vi "TC110_NoFGV.vi"(7 "Function":T3=enum."Read command", 8 "Error in":errorcluster, 10 "Settings in":T2) -> (0 "Error out":errorcluster, 1 "Status_string":string, 2 "Settings out":T2, 3 "output cluster":T1)   [LabVIEW 2018]
uses:
  Ctl/Function_of_TC110.ctl
  PublicSubVI/Ctl/_ctl_RT_TurboSettings.ctl
  Example/RS485_TurboPump/Public/Turbopumps/PV Operating adjustment - Cluster.ctl
  Example/RS485_TurboPump/Pfeiffer Vacuum.lvlib
panel:
  in  "VISA session":refnum<visa-resource-name>
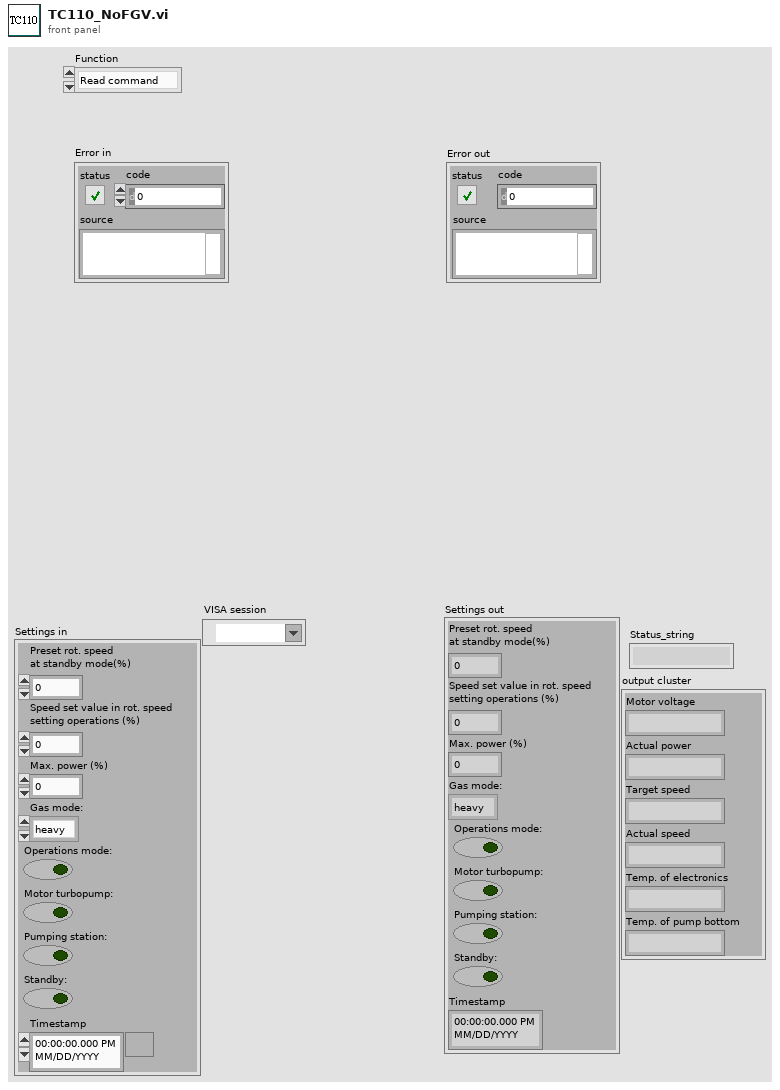
[diagram p1: front panel]
types:
  T1 = cluster{"Motor voltage":string, "Actual power":string, "Target speed":string, "Actual speed":string, "Temp. of electronics":string, "Temp. of pump bottom":string}
  T2 = typedef "_ctl_RT_TurboSettings.ctl" = cluster{"Preset rot. speed \nat standby mode(%)":dbl, "Speed set value in rot. speed \nsetting operations (%)":dbl, "Max. power (%)":dbl, "Gas mode: ":enum16{"heavy", "light", "helium"}, "Operations mode: ":bool, "Motor turbopump: ":bool, "Pumping station: ":bool, "Standby: ":bool, "Timestamp":timestamp}
  T3 = typedef "Function_of_TC110.ctl" = enum16{"Initialisation", "Read status", "Write command", "Read command"}
  T4 = typedef "Pfeiffer Vacuum.lvlib/PV Operating adjustment - Cluster.ctl" = cluster{"Parameter":u16, "Parameter\nread only<->describe":bool, "off<->on":bool, "Rotation speed set value\nin rot. speed setting\noperations [%]":dbl, "Preset rotation Speed\nat Standby mode (%)":dbl, "maximum power\nsetpoint [%]":i32, "Gas mode":u16}
  T5 = enum16{"temperature inverter [°C] (324)", "temperature electronic [°C] (326)", "temperature pump bottom [°C] (330)", "temperature bearing [°C] (342)", "temperature motor [°C] (346)", "temperature rotor [°C] (384)"}
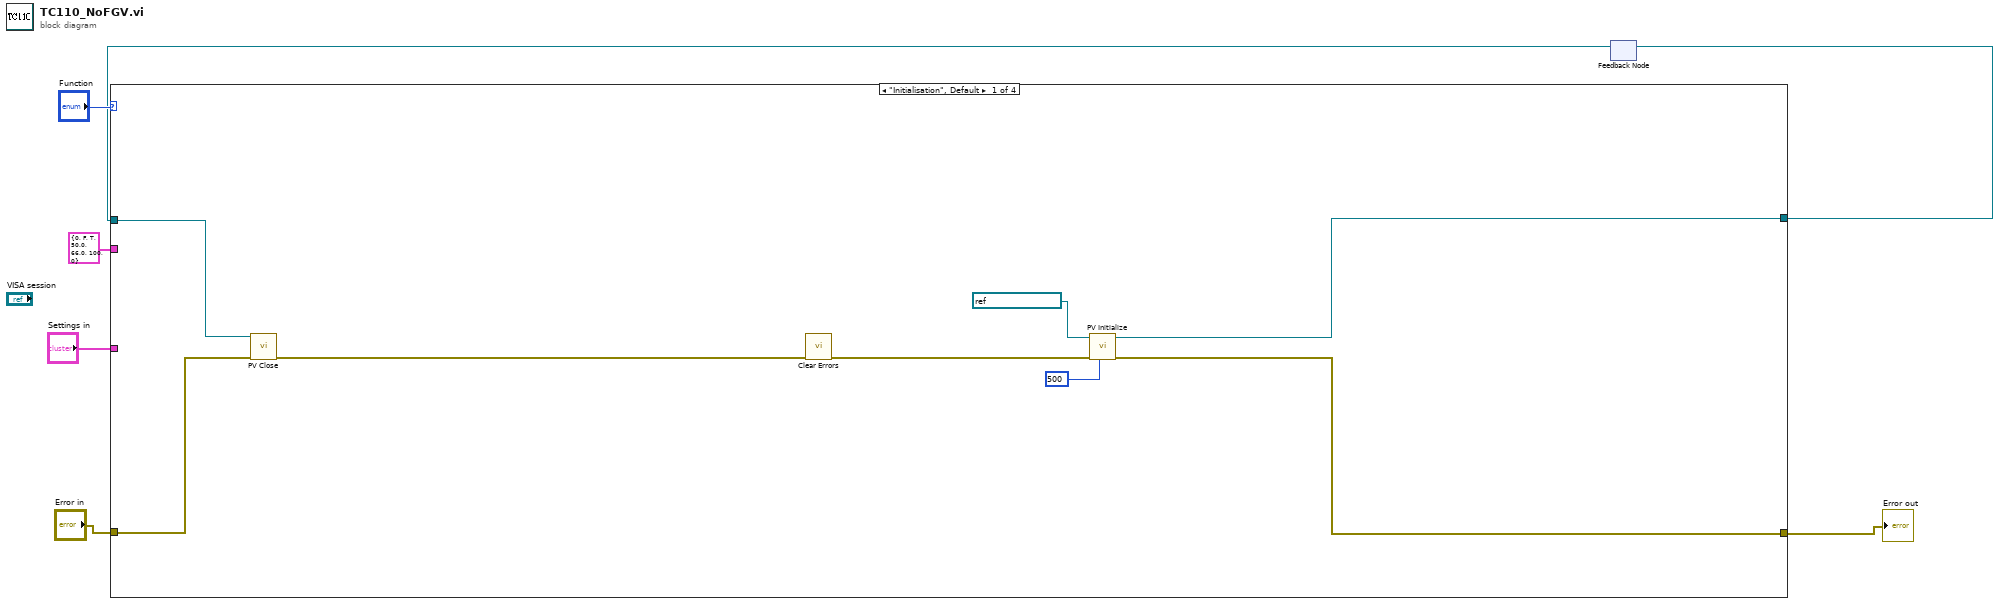
[diagram p0: block diagram]
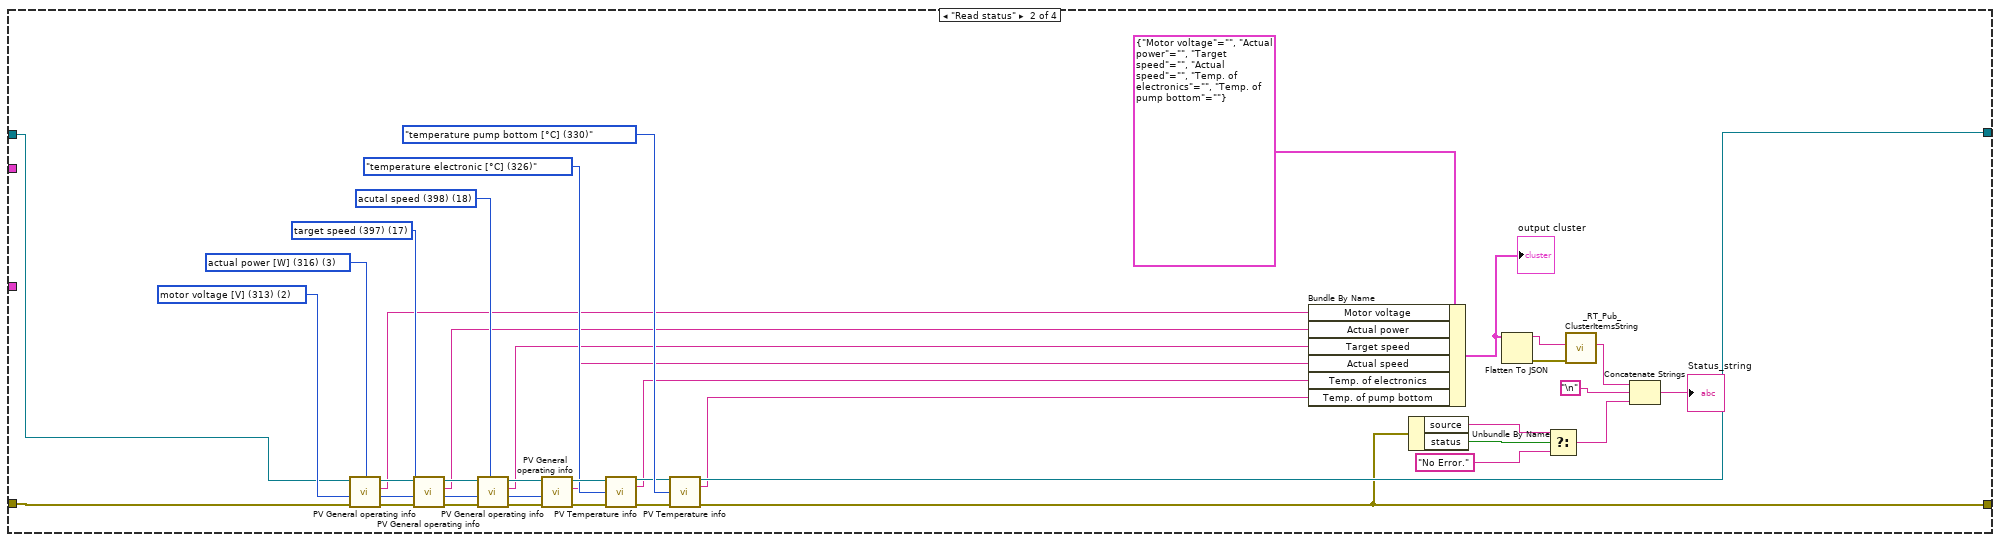
[diagram p2: hidden frame]
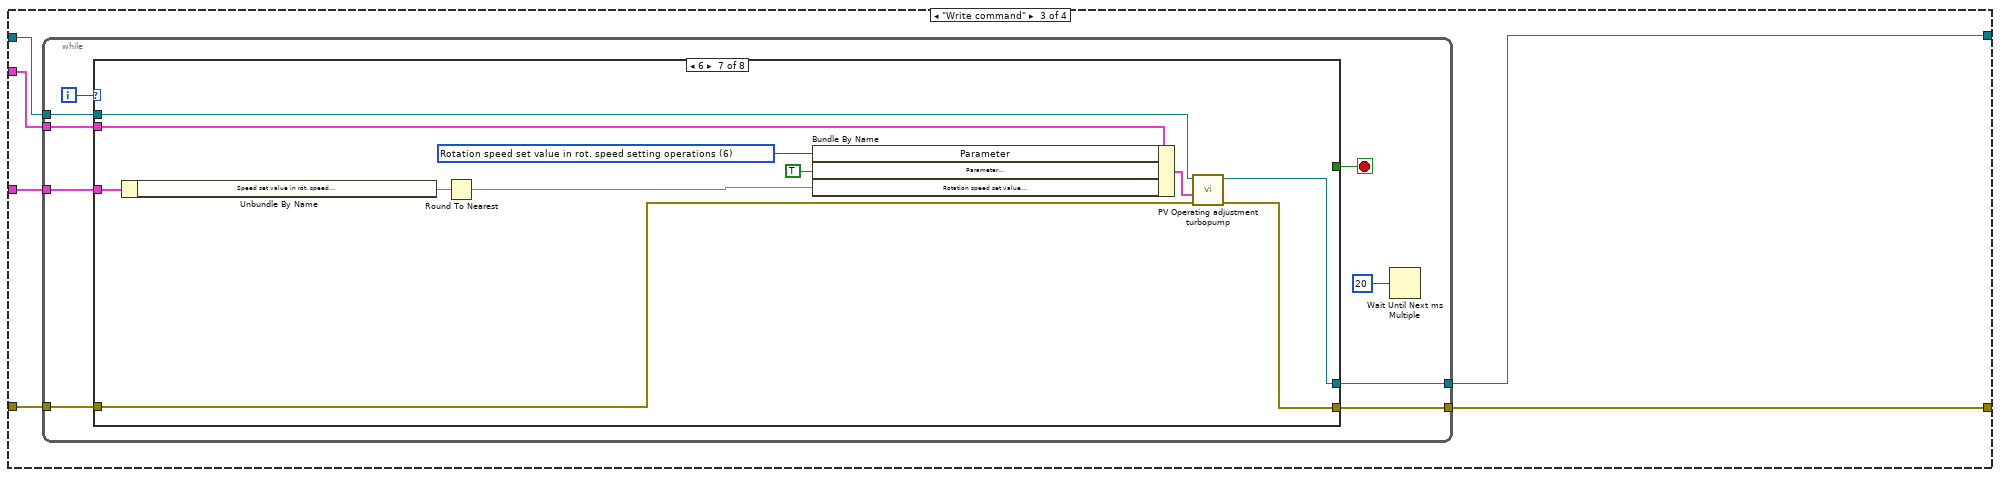
[diagram p3: hidden frame]
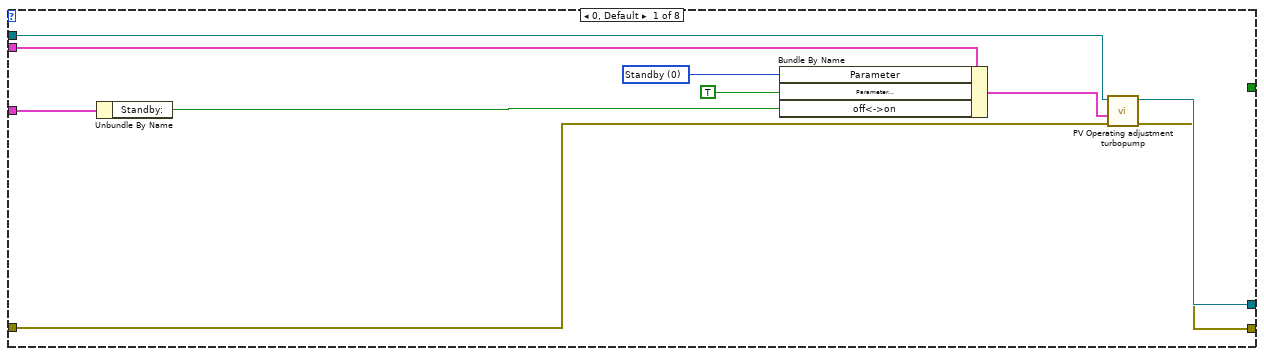
[diagram p4: hidden frame]
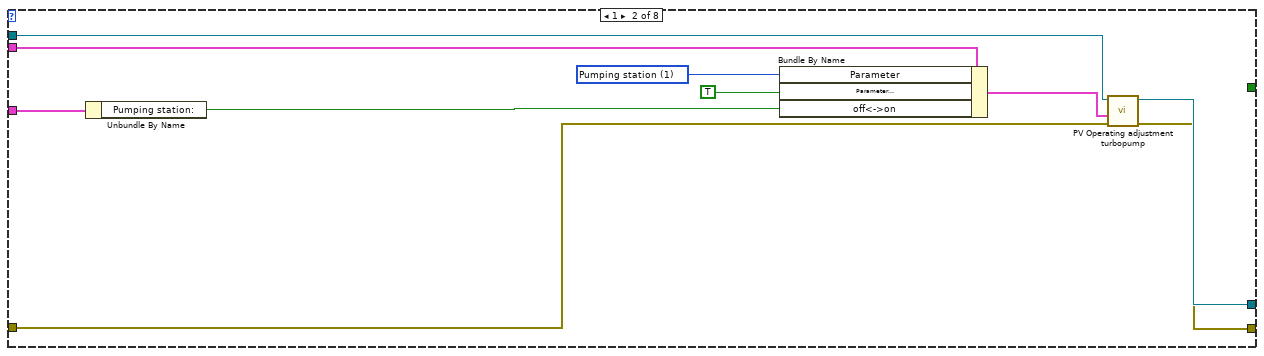
[diagram p5: hidden frame]
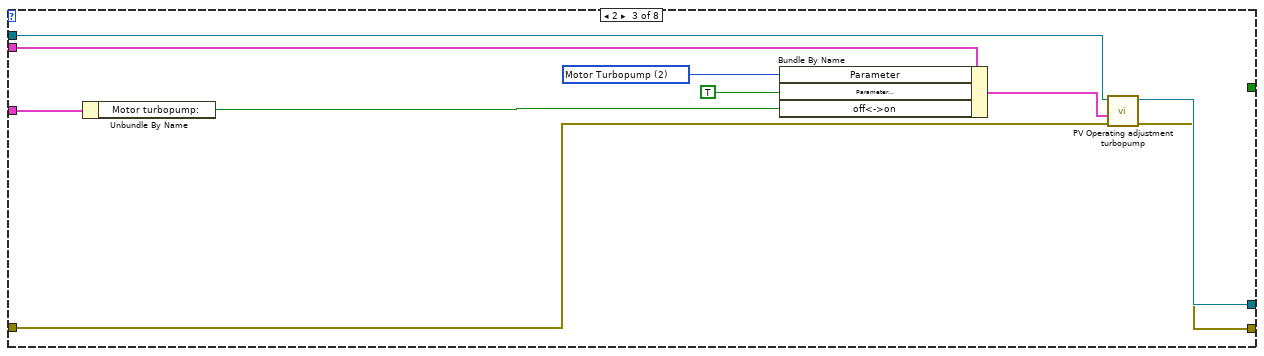
[diagram p6: hidden frame]
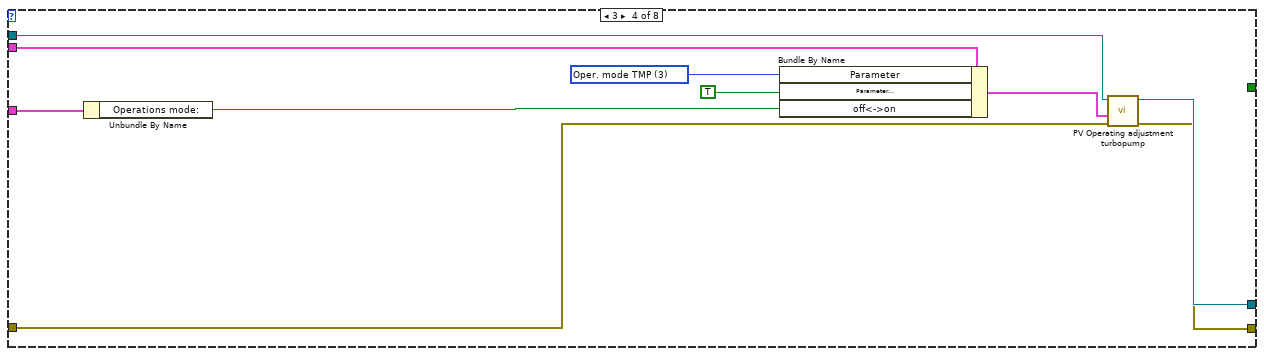
[diagram p7: hidden frame]
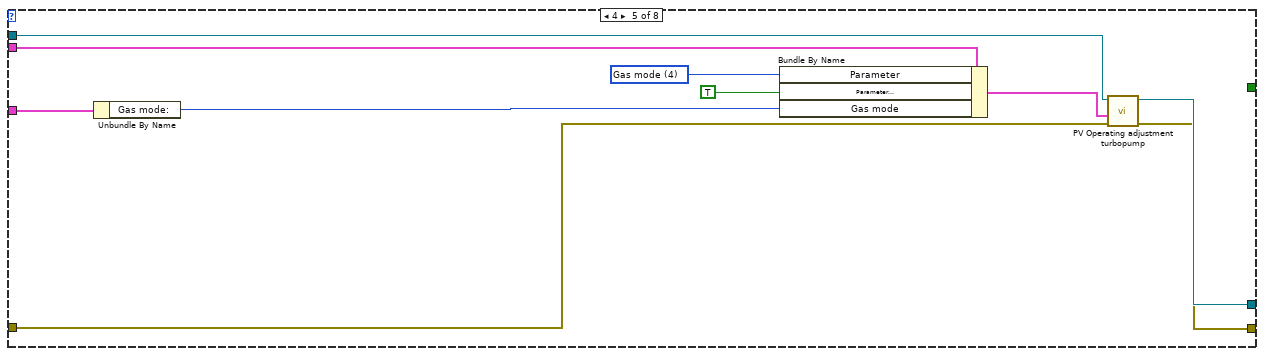
[diagram p8: hidden frame]
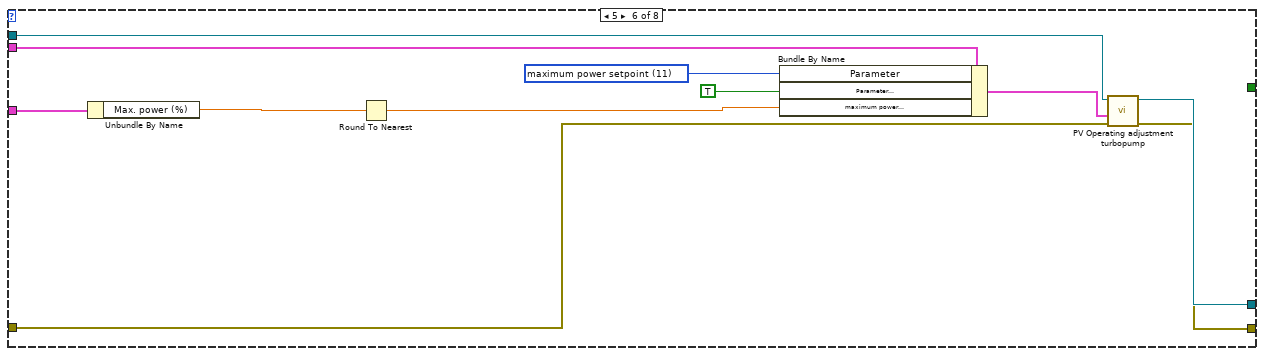
[diagram p9: hidden frame]
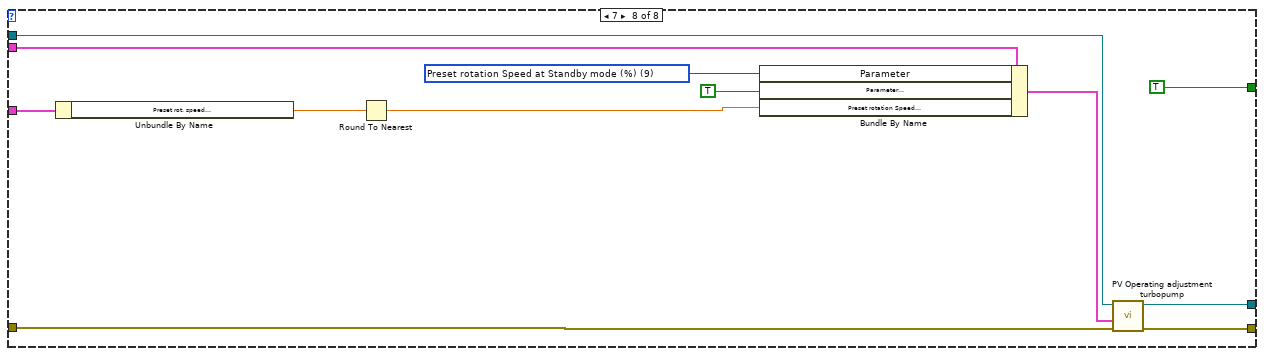
[diagram p10: hidden frame]
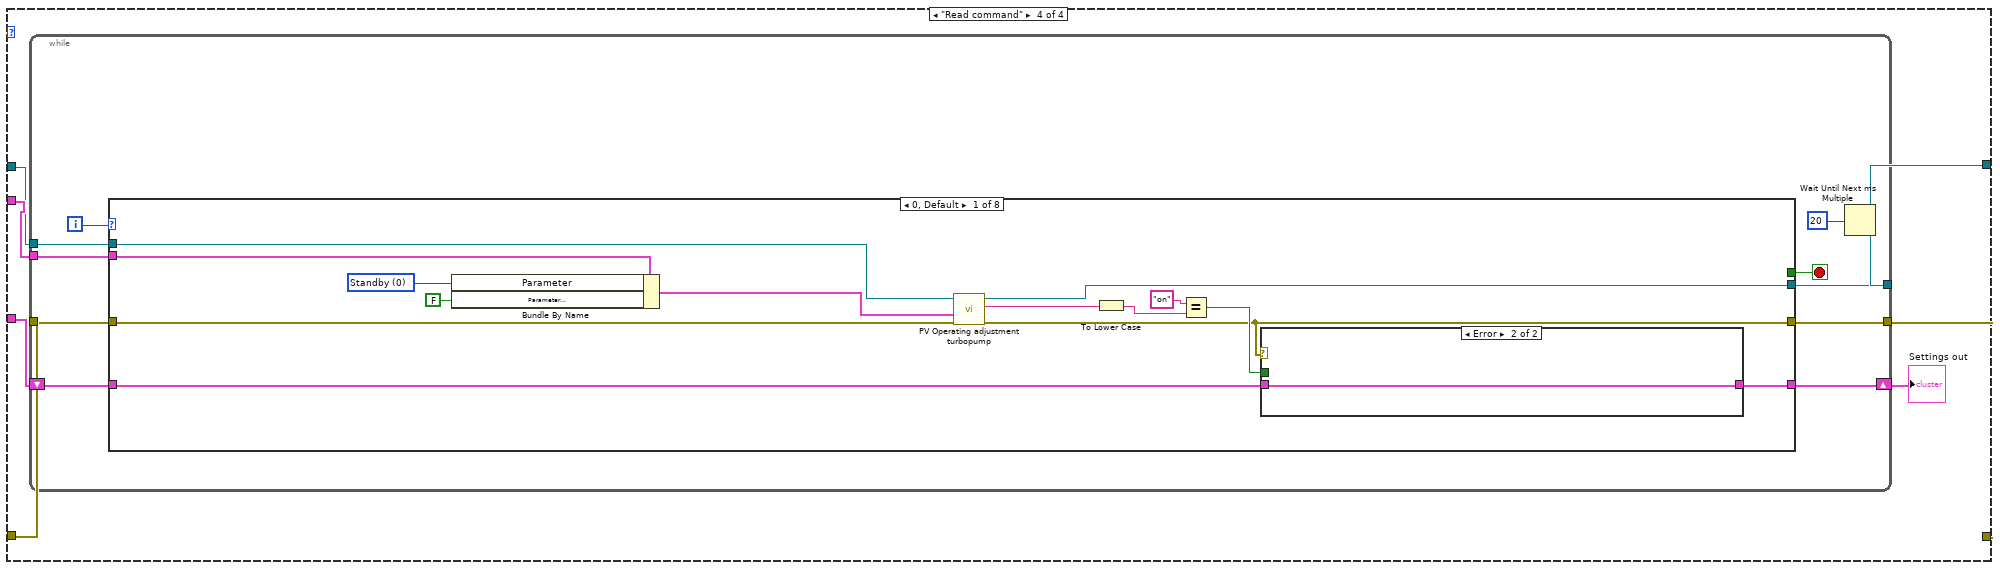
[diagram p11: hidden frame]
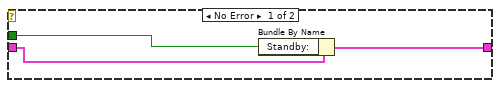
[diagram p12: hidden frame]
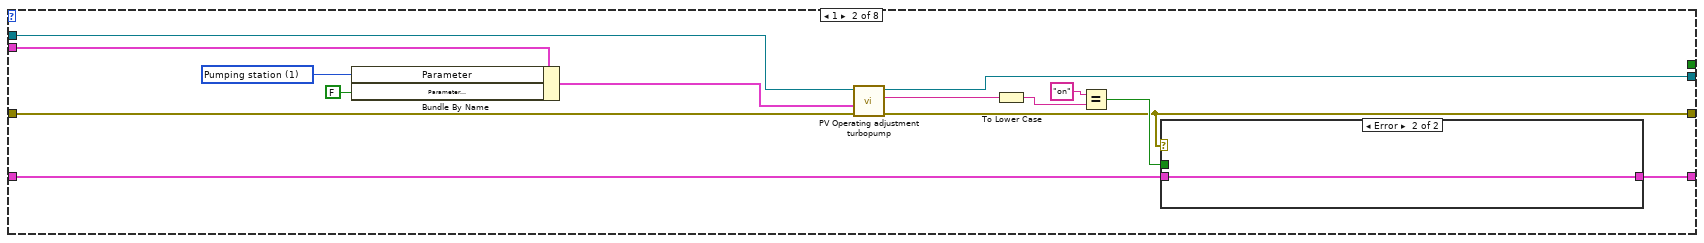
[diagram p13: hidden frame]
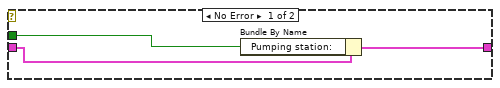
[diagram p14: hidden frame]
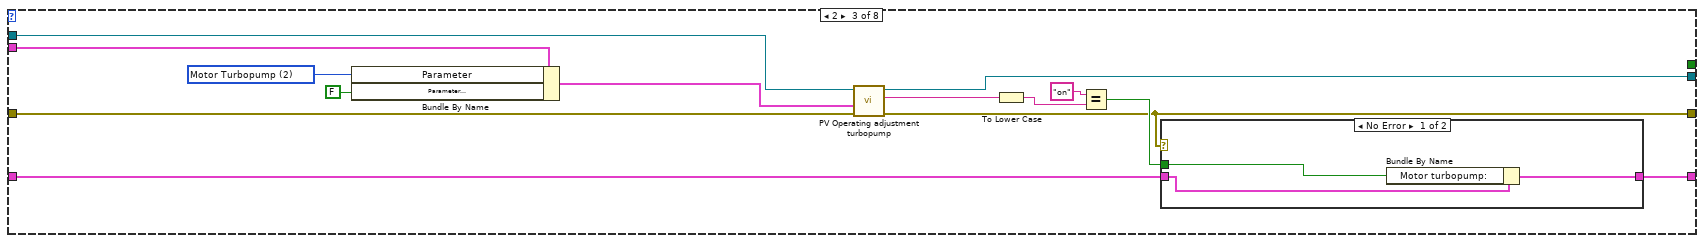
[diagram p15: hidden frame]
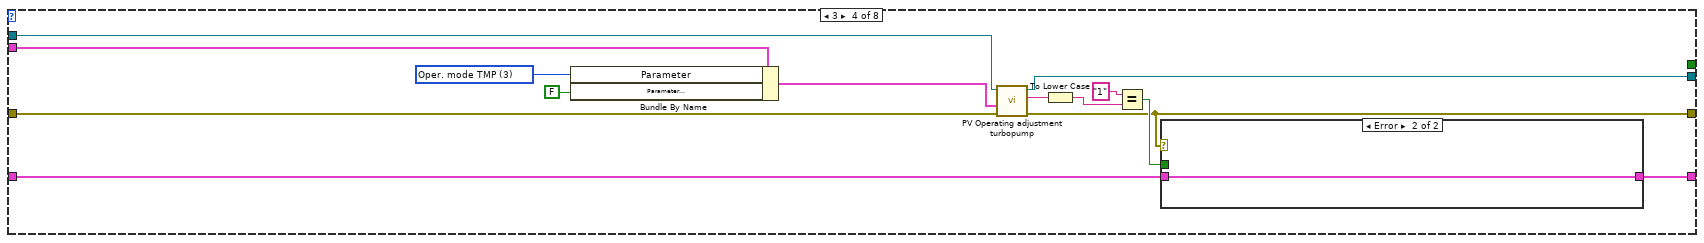
[diagram p17: hidden frame]
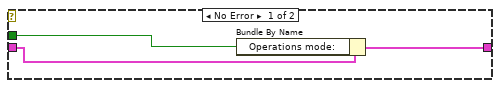
[diagram p18: hidden frame]
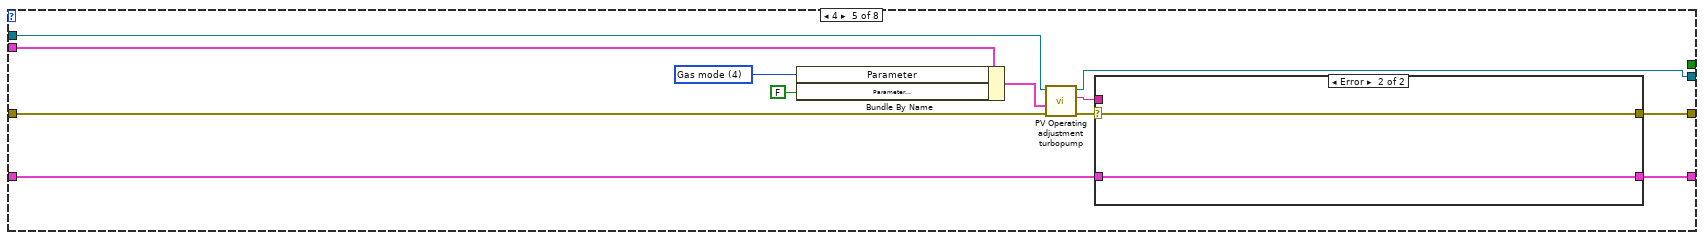
[diagram p19: hidden frame]
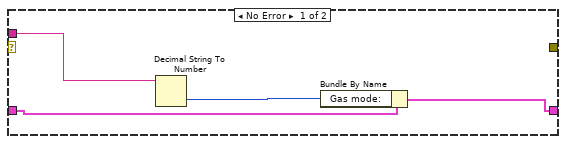
[diagram p20: hidden frame]
diagram:
  n1 = feedback #1() -> (w4:refnum<visa-resource-name>)  [unwired: 1 in]
  n2 = case shown="\"Initialisation\", Default" "Function" {
    tunnel: "Error in" -> [w11 w16 w55 w154]
    tunnel: [w14 w32 w54 w158] -> w5
    tunnel: w4 -> [w12 w17 w56 w155]
    tunnel: [w13 w25 w53 w157] -> w3
    tunnel: "Settings in" -> [_ _ w58 w153]
    tunnel: T4 {"Parameter"=0, "Parameter\nread only<->describe"=FALSE, "off<->on"=TRUE, "Rotation speed set value\nin rot. speed setting\noperations [%]"=50.0, "Preset rotation Speed\nat Standby mode (%)"=66.0, "maximum power\nsetpoint [%]"=100, "Gas mode"=0} ("Operating adjustment - Cluster") -> [_ _ w57 w156]
    frame "Initialisation", Default {
      n3 = call "PV Close.vi"("VISA session"=w12, "error in (no error)"=w11) -> ("error out"=w10:errorcluster)  [unwired: 13 in]
      n4 = call <vilib>:"Clear Errors.vi"("error in (no error)"=w10) -> ("error out"=w9:errorcluster)  [unwired: 5 in, 1 out]
      n5 = call "PV Initialize.vi"("Timeout Value"=u32 500, "error in (no error)"=w9, "VISA session in"=refnum<visa-resource-name> "ASRL3::INSTR") -> ("error out"=w13:errorcluster, "VISA session out"=w14:refnum<visa-resource-name>)  [unwired: 7 in]
    }
    frame "Read status" {
      w48 = u16 18 items=["nominal speed [Hz] (default) (315)", "intermediate circut current [A] (310)", "motor voltage [V] (313)", "actual power [W] (316)", "operating hours pump [h] (311)", "operating hours drive [h] (314)", "pump cycles (read only) (319)", "status oil sensor (read only) (301)", "speed switchpoint attained (read only) (302)", "overtemperature drive (read only) (304)", "overtemperature pump (read only) (305)", "target speed attained (read only) (306)", "pump accelerates (read only) (307) ", "controlled by remote (300)", "motor phase current [A] (317)", "acceleration / deceleration [rm/s] (336)", "hardware version controller (354)", "target speed (397)", "acutal speed (398)", "nominal speed (399)", "software version control unit (read only) (352)"] ("Parameter")
      w49 = u16 17 items=["nominal speed [Hz] (default) (315)", "intermediate circut current [A] (310)", "motor voltage [V] (313)", "actual power [W] (316)", "operating hours pump [h] (311)", "operating hours drive [h] (314)", "pump cycles (read only) (319)", "status oil sensor (read only) (301)", "speed switchpoint attained (read only) (302)", "overtemperature drive (read only) (304)", "overtemperature pump (read only) (305)", "target speed attained (read only) (306)", "pump accelerates (read only) (307) ", "controlled by remote (300)", "motor phase current [A] (317)", "acceleration / deceleration [rm/s] (336)", "hardware version controller (354)", "target speed (397)", "acutal speed (398)", "nominal speed (399)", "software version control unit (read only) (352)"] ("Parameter")
      w50 = u16 3 items=["nominal speed [Hz] (default) (315)", "intermediate circut current [A] (310)", "motor voltage [V] (313)", "actual power [W] (316)", "operating hours pump [h] (311)", "operating hours drive [h] (314)", "pump cycles (read only) (319)", "status oil sensor (read only) (301)", "speed switchpoint attained (read only) (302)", "overtemperature drive (read only) (304)", "overtemperature pump (read only) (305)", "target speed attained (read only) (306)", "pump accelerates (read only) (307) ", "controlled by remote (300)", "motor phase current [A] (317)", "acceleration / deceleration [rm/s] (336)", "hardware version controller (354)", "target speed (397)", "acutal speed (398)", "nominal speed (399)", "software version control unit (read only) (352)"] ("Parameter")
      w52 = u16 2 items=["nominal speed [Hz] (default) (315)", "intermediate circut current [A] (310)", "motor voltage [V] (313)", "actual power [W] (316)", "operating hours pump [h] (311)", "operating hours drive [h] (314)", "pump cycles (read only) (319)", "status oil sensor (read only) (301)", "speed switchpoint attained (read only) (302)", "overtemperature drive (read only) (304)", "overtemperature pump (read only) (305)", "target speed attained (read only) (306)", "pump accelerates (read only) (307) ", "controlled by remote (300)", "motor phase current [A] (317)", "acceleration / deceleration [rm/s] (336)", "hardware version controller (354)", "target speed (397)", "acutal speed (398)", "nominal speed (399)", "software version control unit (read only) (352)"] ("Parameter")
      n6 = call "PV General operating info.vi"("error in (no error)"=w16, "Parameter"=w52, "VISA session"=w17) -> ("error out"=w45:errorcluster, "response (data)"=w35:string, "dup VISA session"=w51:refnum<visa-resource-name>)  [unwired: 6 in]
      n7 = call "PV General operating info.vi"("error in (no error)"=w45, "Parameter"=w50, "VISA session"=w51) -> ("error out"=w44:errorcluster, "response (data)"=w29:string, "dup VISA session"=w47:refnum<visa-resource-name>)  [unwired: 6 in]
      n8 = call "PV General operating info.vi"("error in (no error)"=w44, "Parameter"=w49, "VISA session"=w47) -> ("error out"=w43:errorcluster, "response (data)"=w30:string, "dup VISA session"=w46:refnum<visa-resource-name>)  [unwired: 6 in]
      n9 = call "PV General operating info.vi"("error in (no error)"=w43, "Parameter"=w48, "VISA session"=w46) -> ("error out"=w39:errorcluster, "response (data)"=w34:string, "dup VISA session"=w42:refnum<visa-resource-name>)  [unwired: 6 in]
      n10 = call "PV Temperature info.vi"("VISA session"=w42, "Parameter"=T5."temperature electronic [°C] (326)", "error in (no error)"=w39) -> ("dup VISA session"=w38:refnum<visa-resource-name>, "response (data)"=w33:string, "error out"=w37:errorcluster)  [unwired: 10 in]
      n11 = call "PV Temperature info.vi"("VISA session"=w38, "Parameter"=T5."temperature pump bottom [°C] (330)", "error in (no error)"=w37) -> ("dup VISA session"=w32:refnum<visa-resource-name>, "response (data)"=w31:string, "error out"=w25:errorcluster)  [unwired: 10 in]
      n12 = Bundle By Name(cluster=T1 {"Motor voltage"="", "Actual power"="", "Target speed"="", "Actual speed"="", "Temp. of electronics"="", "Temp. of pump bottom"=""}, "Motor voltage"=w35, "Actual power"=w29, "Target speed"=w30, "Actual speed"=w34, "Temp. of electronics"=w33, "Temp. of pump bottom"=w31) -> (w28:T1)
      "output cluster" <- w28
      n13 = Unbundle By Name(w25) -> ("source"=w23:string, "status"=w24:bool)
      n14 = Flatten To JSON(anything=w28) -> (JSON string=w27:string, 11:w26:errorcluster)  [unwired: 2 in]
      n15 = Select(t=w23, s=w24, f="No Error.") -> (s? t:f=w19:string)
      n16 = call "_RT_Pub_ClusterItemsString.vi"("error in (no error)"=w26, "JSON string"=w27) -> ("result string"=w21:string)  [unwired: 8 in, 1 out]
      n17 = Concatenate Strings(w21, "\n" ("string"), w19) -> (→"Status_string":string)
    }
    frame "Write command" {
      n18 = while {
        tunnel: w58 -> [w67]
        tunnel: w56 -> [w63]
        tunnel: w55 -> [w61]
        tunnel: [w64] -> w54
        tunnel: [w62] -> w53
        tunnel: w57 -> [w66]
        i -> [w65]
        stop <- w60 stop-if-true
        n19 = case shown="6" w65 {
          tunnel: w67 -> [w75 w85 w95 w105 w115 w126 w137 w149]
          tunnel: w66 -> [w77 w87 w97 w107 w117 w128 w139 w151]
          tunnel: [w73 w83 w93 w103 w113 w124 w135 w147] -> w64
          tunnel: w63 -> [w72 w82 w92 w102 w112 w123 w134 w146]
          tunnel: [w70 w80 w90 w100 w110 w121 w132 w145] -> w62
          tunnel: w61 -> [w69 w79 w89 w99 w109 w120 w131 w144]
          tunnel: [_ _ _ _ _ _ _ TRUE] -> w60
          frame 0, Default {
            w68 = u16 0 items=[" Standby", " Pumping station", " Motor Turbopump", " Oper. mode TMP", " Gas mode", " Operating mode drive unit", " Rotation speed set value in rot. speed setting operations", " Set rotation speed TMP [Hz] (read only)", " Actual rotation speed TMP [Hz] (read only)", " Preset rotation Speed at Standby mode (%)", " Max. rotations speed ", " maximum power setpoint"] ("Parameter")
            n20 = Unbundle By Name(w75) -> ("Standby:"=w74:bool)
            n21 = Bundle By Name(cluster=w77, "Parameter"=w68, "Parameter\nread only<->describe"=TRUE ("Parameter\nread only<->describe"), "off<->on"=w74) -> (w71:T4)
            n22 = call "PV Operating adjustment turbopump.vi"("error in (no error)"=w69, "Operating adjustment - Cluster"=w71, "VISA session"=w72) -> ("error out"=w70:errorcluster, "dup VISA session"=w73:refnum<visa-resource-name>)  [unwired: 6 in, 1 out]
          }
          frame 1 {
            w78 = u16 1 items=[" Standby", " Pumping station", " Motor Turbopump", " Oper. mode TMP", " Gas mode", " Operating mode drive unit", " Rotation speed set value in rot. speed setting operations", " Set rotation speed TMP [Hz] (read only)", " Actual rotation speed TMP [Hz] (read only)", " Preset rotation Speed at Standby mode (%)", " Max. rotations speed ", " maximum power setpoint"] ("Parameter")
            n23 = Unbundle By Name(w85) -> ("Pumping station:"=w84:bool)
            n24 = Bundle By Name(cluster=w87, "Parameter"=w78, "Parameter\nread only<->describe"=TRUE ("Parameter\nread only<->describe"), "off<->on"=w84) -> (w81:T4)
            n25 = call "PV Operating adjustment turbopump.vi"("error in (no error)"=w79, "Operating adjustment - Cluster"=w81, "VISA session"=w82) -> ("error out"=w80:errorcluster, "dup VISA session"=w83:refnum<visa-resource-name>)  [unwired: 6 in, 1 out]
          }
          frame 2 {
            w88 = u16 2 items=[" Standby", " Pumping station", " Motor Turbopump", " Oper. mode TMP", " Gas mode", " Operating mode drive unit", " Rotation speed set value in rot. speed setting operations", " Set rotation speed TMP [Hz] (read only)", " Actual rotation speed TMP [Hz] (read only)", " Preset rotation Speed at Standby mode (%)", " Max. rotations speed ", " maximum power setpoint"] ("Parameter")
            n26 = Unbundle By Name(w95) -> ("Motor turbopump:"=w94:bool)
            n27 = Bundle By Name(cluster=w97, "Parameter"=w88, "Parameter\nread only<->describe"=TRUE ("Parameter\nread only<->describe"), "off<->on"=w94) -> (w91:T4)
            n28 = call "PV Operating adjustment turbopump.vi"("error in (no error)"=w89, "Operating adjustment - Cluster"=w91, "VISA session"=w92) -> ("error out"=w90:errorcluster, "dup VISA session"=w93:refnum<visa-resource-name>)  [unwired: 6 in, 1 out]
          }
          frame 3 {
            w98 = u16 3 items=[" Standby", " Pumping station", " Motor Turbopump", " Oper. mode TMP", " Gas mode", " Operating mode drive unit", " Rotation speed set value in rot. speed setting operations", " Set rotation speed TMP [Hz] (read only)", " Actual rotation speed TMP [Hz] (read only)", " Preset rotation Speed at Standby mode (%)", " Max. rotations speed ", " maximum power setpoint"] ("Parameter")
            n29 = Unbundle By Name(w105) -> ("Operations mode:"=w104:bool)
            n30 = Bundle By Name(cluster=w107, "Parameter"=w98, "Parameter\nread only<->describe"=TRUE ("Parameter\nread only<->describe"), "off<->on"=w104) -> (w101:T4)
            n31 = call "PV Operating adjustment turbopump.vi"("error in (no error)"=w99, "Operating adjustment - Cluster"=w101, "VISA session"=w102) -> ("error out"=w100:errorcluster, "dup VISA session"=w103:refnum<visa-resource-name>)  [unwired: 6 in, 1 out]
          }
          frame 4 {
            w108 = u16 4 items=[" Standby", " Pumping station", " Motor Turbopump", " Oper. mode TMP", " Gas mode", " Operating mode drive unit", " Rotation speed set value in rot. speed setting operations", " Set rotation speed TMP [Hz] (read only)", " Actual rotation speed TMP [Hz] (read only)", " Preset rotation Speed at Standby mode (%)", " Max. rotations speed ", " maximum power setpoint"] ("Parameter")
            n32 = Unbundle By Name(w115) -> ("Gas mode:"=w114:enum16{"heavy", "light", "helium"})
            n33 = Bundle By Name(cluster=w117, "Parameter"=w108, "Parameter\nread only<->describe"=TRUE ("Parameter\nread only<->describe"), "Gas mode"=w114) -> (w111:T4)
            n34 = call "PV Operating adjustment turbopump.vi"("error in (no error)"=w109, "Operating adjustment - Cluster"=w111, "VISA session"=w112) -> ("error out"=w110:errorcluster, "dup VISA session"=w113:refnum<visa-resource-name>)  [unwired: 6 in, 1 out]
          }
          frame 5 {
            w119 = u16 11 items=[" Standby", " Pumping station", " Motor Turbopump", " Oper. mode TMP", " Gas mode", " Operating mode drive unit", " Rotation speed set value in rot. speed setting operations", " Set rotation speed TMP [Hz] (read only)", " Actual rotation speed TMP [Hz] (read only)", " Preset rotation Speed at Standby mode (%)", " Max. rotations speed ", " maximum power setpoint"] ("Parameter")
            n35 = Unbundle By Name(w126) -> ("Max. power (%)"=w125:dbl)
            n36 = Round To Nearest(number=w125) -> (nearest integer value=w118:dbl)
            n37 = Bundle By Name(cluster=w128, "Parameter"=w119, "Parameter\nread only<->describe"=TRUE ("Parameter\nread only<->describe"), "maximum power\nsetpoint [%]"=w118) -> (w122:T4)
            n38 = call "PV Operating adjustment turbopump.vi"("error in (no error)"=w120, "Operating adjustment - Cluster"=w122, "VISA session"=w123) -> ("error out"=w121:errorcluster, "dup VISA session"=w124:refnum<visa-resource-name>)  [unwired: 6 in, 1 out]
          }
          frame 6 {
            w130 = u16 6 items=[" Standby", " Pumping station", " Motor Turbopump", " Oper. mode TMP", " Gas mode", " Operating mode drive unit", " Rotation speed set value in rot. speed setting operations", " Set rotation speed TMP [Hz] (read only)", " Actual rotation speed TMP [Hz] (read only)", " Preset rotation Speed at Standby mode (%)", " Max. rotations speed ", " maximum power setpoint"] ("Parameter")
            n39 = Unbundle By Name(w137) -> ("Speed set value in rot. speed \nsetting operations (%)"=w136:dbl)
            n40 = Round To Nearest(number=w136) -> (nearest integer value=w129:dbl)
            n41 = Bundle By Name(cluster=w139, "Parameter"=w130, "Parameter\nread only<->describe"=TRUE ("Parameter\nread only<->describe"), "Rotation speed set value\nin rot. speed setting\noperations [%]"=w129) -> (w133:T4)
            n42 = call "PV Operating adjustment turbopump.vi"("error in (no error)"=w131, "Operating adjustment - Cluster"=w133, "VISA session"=w134) -> ("error out"=w132:errorcluster, "dup VISA session"=w135:refnum<visa-resource-name>)  [unwired: 6 in, 1 out]
          }
          frame 7 {
            w143 = u16 9 items=[" Standby", " Pumping station", " Motor Turbopump", " Oper. mode TMP", " Gas mode", " Operating mode drive unit", " Rotation speed set value in rot. speed setting operations", " Set rotation speed TMP [Hz] (read only)", " Actual rotation speed TMP [Hz] (read only)", " Preset rotation Speed at Standby mode (%)", " Max. rotations speed ", " maximum power setpoint"] ("Parameter")
            n43 = Unbundle By Name(w149) -> ("Preset rot. speed \nat standby mode(%)"=w148:dbl)
            n44 = Round To Nearest(number=w148) -> (nearest integer value=w142:dbl)
            n45 = Bundle By Name(cluster=w151, "Parameter"=w143, "Parameter\nread only<->describe"=TRUE ("Parameter\nread only<->describe"), "Preset rotation Speed\nat Standby mode (%)"=w142) -> (w141:T4)
            n46 = call "PV Operating adjustment turbopump.vi"("error in (no error)"=w144, "Operating adjustment - Cluster"=w141, "VISA session"=w146) -> ("error out"=w145:errorcluster, "dup VISA session"=w147:refnum<visa-resource-name>)  [unwired: 6 in, 1 out]
          }
        }
        n47 = Wait Until Next ms Multiple(millisecond multiple=u32 20) -> ()  [unwired: 1 out]
      }
    }
    frame "Read command" {
      n48 = while {
        tunnel: w155 -> [w165]
        tunnel: w154 -> [w163]
        tunnel: [w166] -> w158
        tunnel: [w164] -> w157
        shift-right: [w160] -> w152
        shift-left: w153 -> [w161]
        tunnel: w156 -> [w168]
        i -> [w167]
        stop <- w162 stop-if-true
        n49 = case shown="0, Default" w167 {
          tunnel: w168 -> [w173 w200 w218 w236 w252 w270 w287 w304]
          tunnel: [w181 w198 w216 w234 w250 w268 w285 w302] -> w166
          tunnel: w165 -> [w180 w197 w215 w233 w249 w267 w284 w301]
          tunnel: [w169 w187 w205 w223 w241 w259 w280 w296] -> w164
          tunnel: w163 -> [w178 w195 w213 w231 w247 w266 w282 w300]
          tunnel: [_ _ _ _ _ _ _ TRUE] -> w162
          tunnel: w161 -> [w172 w189 w207 w224 w244 w262 w278 w295]
          tunnel: [w170 w190 w206 w225 w243 w261 w277 w294] -> w160
          frame 0, Default {
            w177 = u16 0 items=[" Standby", " Pumping station", " Motor Turbopump", " Oper. mode TMP", " Gas mode", " Operating mode drive unit", " Rotation speed set value in rot. speed setting operations", " Set rotation speed TMP [Hz] (read only)", " Actual rotation speed TMP [Hz] (read only)", " Preset rotation Speed at Standby mode (%)", " Max. rotations speed ", " maximum power setpoint"] ("Parameter")
            n50 = Bundle By Name(cluster=w173, "Parameter"=w177, "Parameter\nread only<->describe"=FALSE ("Parameter\nread only<->describe")) -> (w179:T4)
            n51 = call "PV Operating adjustment turbopump.vi"("error in (no error)"=w178, "Operating adjustment - Cluster"=w179, "VISA session"=w180) -> ("error out"=w169:errorcluster, "response (data)"=w174:string, "dup VISA session"=w181:refnum<visa-resource-name>)  [unwired: 6 in]
            n52 = To Lower Case(string=w174) -> (all lower case string=w175:string)
            n53 = Equal?(x="on", y=w175) -> (x = y?=w171:bool)
            n54 = case shown="Error" w169 {
              tunnel: w172 -> [w185 w186]
              tunnel: w171 -> [w184 _]
              tunnel: [w183 w186] -> w170
              frame No Error {
                n55 = Bundle By Name(cluster=w185, "Standby:"=w184) -> (w183:T2)
              }
              frame Error {
              }
            }
          }
          frame 1 {
            w194 = u16 1 items=[" Standby", " Pumping station", " Motor Turbopump", " Oper. mode TMP", " Gas mode", " Operating mode drive unit", " Rotation speed set value in rot. speed setting operations", " Set rotation speed TMP [Hz] (read only)", " Actual rotation speed TMP [Hz] (read only)", " Preset rotation Speed at Standby mode (%)", " Max. rotations speed ", " maximum power setpoint"] ("Parameter")
            n56 = Bundle By Name(cluster=w200, "Parameter"=w194, "Parameter\nread only<->describe"=FALSE ("Parameter\nread only<->describe")) -> (w196:T4)
            n57 = call "PV Operating adjustment turbopump.vi"("error in (no error)"=w195, "Operating adjustment - Cluster"=w196, "VISA session"=w197) -> ("error out"=w187:errorcluster, "response (data)"=w188:string, "dup VISA session"=w198:refnum<visa-resource-name>)  [unwired: 6 in]
            n58 = To Lower Case(string=w188) -> (all lower case string=w192:string)
            n59 = Equal?(x="on", y=w192) -> (x = y?=w191:bool)
            n60 = case shown="Error" w187 {
              tunnel: w191 -> [w203 _]
              tunnel: [w202 w204] -> w190
              tunnel: w189 -> [w201 w204]
              frame No Error {
                n61 = Bundle By Name(cluster=w201, "Pumping station:"=w203) -> (w202:T2)
              }
              frame Error {
              }
            }
          }
          frame 2 {
            w212 = u16 2 items=[" Standby", " Pumping station", " Motor Turbopump", " Oper. mode TMP", " Gas mode", " Operating mode drive unit", " Rotation speed set value in rot. speed setting operations", " Set rotation speed TMP [Hz] (read only)", " Actual rotation speed TMP [Hz] (read only)", " Preset rotation Speed at Standby mode (%)", " Max. rotations speed ", " maximum power setpoint"] ("Parameter")
            n62 = Bundle By Name(cluster=w218, "Parameter"=w212, "Parameter\nread only<->describe"=FALSE ("Parameter\nread only<->describe")) -> (w214:T4)
            n63 = call "PV Operating adjustment turbopump.vi"("error in (no error)"=w213, "Operating adjustment - Cluster"=w214, "VISA session"=w215) -> ("error out"=w205:errorcluster, "response (data)"=w208:string, "dup VISA session"=w216:refnum<visa-resource-name>)  [unwired: 6 in]
            n64 = To Lower Case(string=w208) -> (all lower case string=w210:string)
            n65 = Equal?(x="on", y=w210) -> (x = y?=w209:bool)
            n66 = case shown="No Error" w205 {
              tunnel: w209 -> [w221 _]
              tunnel: w207 -> [w220 w222]
              tunnel: [w219 w222] -> w206
              frame No Error {
                n67 = Bundle By Name(cluster=w220, "Motor turbopump:"=w221) -> (w219:T2)
              }
              frame Error {
              }
            }
          }
          frame 3 {
            w230 = u16 3 items=[" Standby", " Pumping station", " Motor Turbopump", " Oper. mode TMP", " Gas mode", " Operating mode drive unit", " Rotation speed set value in rot. speed setting operations", " Set rotation speed TMP [Hz] (read only)", " Actual rotation speed TMP [Hz] (read only)", " Preset rotation Speed at Standby mode (%)", " Max. rotations speed ", " maximum power setpoint"] ("Parameter")
            n68 = Bundle By Name(cluster=w236, "Parameter"=w230, "Parameter\nread only<->describe"=FALSE ("Parameter\nread only<->describe")) -> (w232:T4)
            n69 = call "PV Operating adjustment turbopump.vi"("error in (no error)"=w231, "Operating adjustment - Cluster"=w232, "VISA session"=w233) -> ("error out"=w223:errorcluster, "response (data)"=w226:string, "dup VISA session"=w234:refnum<visa-resource-name>)  [unwired: 6 in]
            n70 = To Lower Case(string=w226) -> (all lower case string=w228:string)
            n71 = Equal?(x="1", y=w228) -> (x = y?=w227:bool)
            n72 = case shown="Error" w223 {
              tunnel: w227 -> [w239 _]
              tunnel: [w238 w240] -> w225
              tunnel: w224 -> [w237 w240]
              frame No Error {
                n73 = Bundle By Name(cluster=w237, "Operations mode:"=w239) -> (w238:T2)
              }
              frame Error {
              }
            }
          }
          frame 4 {
            w246 = u16 4 items=[" Standby", " Pumping station", " Motor Turbopump", " Oper. mode TMP", " Gas mode", " Operating mode drive unit", " Rotation speed set value in rot. speed setting operations", " Set rotation speed TMP [Hz] (read only)", " Actual rotation speed TMP [Hz] (read only)", " Preset rotation Speed at Standby mode (%)", " Max. rotations speed ", " maximum power setpoint"] ("Parameter")
            n74 = Bundle By Name(cluster=w252, "Parameter"=w246, "Parameter\nread only<->describe"=FALSE ("Parameter\nread only<->describe")) -> (w248:T4)
            n75 = call "PV Operating adjustment turbopump.vi"("error in (no error)"=w247, "Operating adjustment - Cluster"=w248, "VISA session"=w249) -> ("error out"=w245:errorcluster, "response (data)"=w242:string, "dup VISA session"=w250:refnum<visa-resource-name>)  [unwired: 6 in]
            n76 = case shown="Error" w245 {
              selector: w245 -> [_ w257]
              tunnel: w244 -> [w256 w258]
              tunnel: w242 -> [w255 _]
              tunnel: [w253 w258] -> w243
              tunnel: [_ w257] -> w241
              frame No Error {
                n77 = Decimal String To Number(string=w255) -> (number=w254:i32)  [unwired: 2 in, 1 out]
                n78 = Bundle By Name(cluster=w256, "Gas mode:"=w254) -> (w253:T2)
              }
              frame Error {
              }
            }
          }
          frame 5 {
            w265 = u16 11 items=[" Standby", " Pumping station", " Motor Turbopump", " Oper. mode TMP", " Gas mode", " Operating mode drive unit", " Rotation speed set value in rot. speed setting operations", " Set rotation speed TMP [Hz] (read only)", " Actual rotation speed TMP [Hz] (read only)", " Preset rotation Speed at Standby mode (%)", " Max. rotations speed ", " maximum power setpoint"] ("Parameter")
            n79 = Bundle By Name(cluster=w270, "Parameter"=w265, "Parameter\nread only<->describe"=FALSE ("Parameter\nread only<->describe")) -> (w264:T4)
            n80 = call "PV Operating adjustment turbopump.vi"("error in (no error)"=w266, "Operating adjustment - Cluster"=w264, "VISA session"=w267) -> ("error out"=w260:errorcluster, "response (data)"=w263:string, "dup VISA session"=w268:refnum<visa-resource-name>)  [unwired: 6 in]
            n81 = case shown="No Error" w260 {
              selector: w260 -> [_ w275]
              tunnel: w263 -> [w273 _]
              tunnel: w262 -> [w272 w276]
              tunnel: [w271 w276] -> w261
              tunnel: [_ w275] -> w259
              frame No Error {
                n82 = Fract/Exp String To Number(string=w273) -> (number=w274:dbl)  [unwired: 3 in, 1 out]
                n83 = Bundle By Name(cluster=w272, "Max. power (%)"=w274) -> (w271:T2)
              }
              frame Error {
              }
            }
          }
          frame 6 {
            w281 = u16 6 items=[" Standby", " Pumping station", " Motor Turbopump", " Oper. mode TMP", " Gas mode", " Operating mode drive unit", " Rotation speed set value in rot. speed setting operations", " Set rotation speed TMP [Hz] (read only)", " Actual rotation speed TMP [Hz] (read only)", " Preset rotation Speed at Standby mode (%)", " Max. rotations speed ", " maximum power setpoint"] ("Parameter")
            n84 = Bundle By Name(cluster=w287, "Parameter"=w281, "Parameter\nread only<->describe"=FALSE ("Parameter\nread only<->describe")) -> (w283:T4)
            n85 = call "PV Operating adjustment turbopump.vi"("error in (no error)"=w282, "Operating adjustment - Cluster"=w283, "VISA session"=w284) -> ("error out"=w280:errorcluster, "response (data)"=w279:string, "dup VISA session"=w285:refnum<visa-resource-name>)  [unwired: 6 in]
            n86 = case shown="No Error" w280 {
              tunnel: w279 -> [w290 _]
              tunnel: w278 -> [w289 w292]
              tunnel: [w288 w292] -> w277
              frame No Error {
                n87 = Fract/Exp String To Number(string=w290) -> (number=w291:dbl)  [unwired: 3 in, 1 out]
                n88 = Bundle By Name(cluster=w289, "Speed set value in rot. speed \nsetting operations (%)"=w291) -> (w288:T2)
              }
              frame Error {
              }
            }
          }
          frame 7 {
            w299 = u16 9 items=[" Standby", " Pumping station", " Motor Turbopump", " Oper. mode TMP", " Gas mode", " Operating mode drive unit", " Rotation speed set value in rot. speed setting operations", " Set rotation speed TMP [Hz] (read only)", " Actual rotation speed TMP [Hz] (read only)", " Preset rotation Speed at Standby mode (%)", " Max. rotations speed ", " maximum power setpoint"] ("Parameter")
            n89 = Bundle By Name(cluster=w304, "Parameter"=w299, "Parameter\nread only<->describe"=FALSE ("Parameter\nread only<->describe")) -> (w298:T4)
            n90 = call "PV Operating adjustment turbopump.vi"("error in (no error)"=w300, "Operating adjustment - Cluster"=w298, "VISA session"=w301) -> ("error out"=w296:errorcluster, "response (data)"=w293:string, "dup VISA session"=w302:refnum<visa-resource-name>)  [unwired: 6 in]
            n91 = case shown="No Error" w296 {
              tunnel: w295 -> [w307 w311]
              tunnel: [w306 w311] -> w294
              tunnel: w293 -> [w305 _]
              frame No Error {
                n92 = Fract/Exp String To Number(string=w305) -> (number=w310:dbl)  [unwired: 3 in, 1 out]
                n93 = Divide(x=w310, y=100.0) -> (x/y=w309:dbl)
                n94 = Bundle By Name(cluster=w307, "Preset rot. speed \nat standby mode(%)"=w309) -> (w306:T2)
              }
              frame Error {
              }
            }
          }
        }
        n95 = Wait Until Next ms Multiple(millisecond multiple=u32 20) -> ()  [unwired: 1 out]
      }
      "Settings out" <- w152
    }
  }
  "Error out" <- w3
  n96 = feedback-in #1(w5) -> ()
